vi "_Config Updated.vi"(8 "error in (no error)":errorcluster, 10 "Config Map":map{string, string}(c390), 11 "DeploySerialResource in":refnum<class "SerialResource.lvclass">) -> (0 "error out":errorcluster, 3 "DeploySerialResource out":refnum<class "SerialResource.lvclass">)   [LabVIEW 2020, in "PicoG-Core.lvlib" / "SerialResource.lvclass"]
uses:
  SerialResource.lvclass
  SerialResource.lvclass/SerialResource.ctl
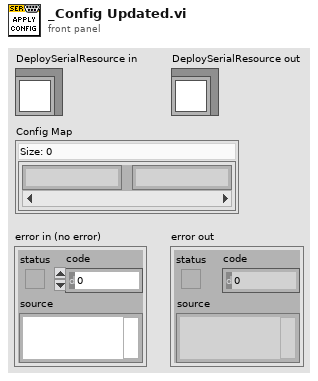
[diagram p1: front panel]
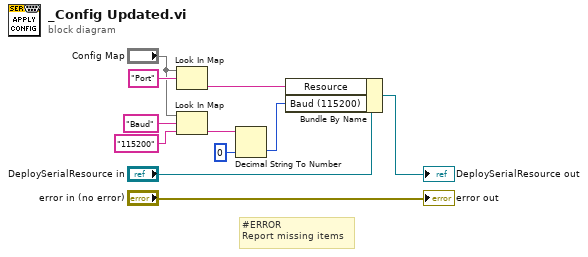
[diagram p0: block diagram]
diagram:
  # "#ERROR\nReport missing items"
  n1 = Look In Map(map="Config Map", key="Port") -> (value=w2:string)  [unwired: 1 in, 1 out]
  n2 = Look In Map(map="Config Map", key="Baud", default value="115200" ("key")) -> (value=w6:string)  [unwired: 1 out]
  n3 = Decimal String To Number(string=w6, default (0L)=u32 0 ("default (0 I32)")) -> (number=w1:u32)  [unwired: 1 in, 1 out]
  n4 = Bundle By Name(cluster="DeploySerialResource in", "Resource"=w2, "Baud (115200)"=w1) -> (→"DeploySerialResource out":refnum<class "SerialResource.lvclass">)
  "error out" <- "error in (no error)"
